vi "0-Load Map.vi"(2 "Map Name":T1="Lake Waban", 3 "Image Ref In":T2) -> (0 "Image Descriptor":T3={"Upper-Left Corner Coordinates"={"UTM Zone"=0.0, "Hemisphere"=enum."North", "East"=0.0, "North"=0.0}, "Meters/Pixel"=1.0} {"Upper-Left Corner Coordinates"."North" format="%#_10f"; "Upper-Left Corner Coordinates"."East" format="%#_8f"}, 1 "Image Ref Out":T2)   [LabVIEW 2011]
doc: "Loads a map and its corresponding descriptor text file.\n\n.png will be added to the given Map Name to get the image,\n.txt will be added to get the image descriptor (The image and the descriptor file have the same filename but different extensions)\nfiles will be retrieved from the /locations/ folder."
uses:
  0-Image Descriptor.ctl
  2-Think/2 Typedefs/UTM Location.ctl
  <vilib>/vision/Image Controls.llb/IMAQ Image.ctl
  0 Typedefs/Maps.ctl
panel:
  # ".png will be added to the map name to get the image,\n.txt will be added to get the image descriptor"
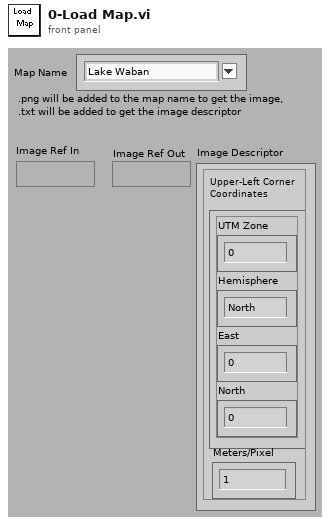
[diagram p1: front panel]
types:
  T1 = typedef "Maps.ctl" = string
  T2 = typedef "IMAQ Image.ctl" = refnum<image>
  T3 = typedef "0-Image Descriptor.ctl" = cluster{"Upper-Left Corner Coordinates":T4, "Meters/Pixel":dbl}
  T4 = typedef "UTM Location.ctl" = cluster{"UTM Zone":dbl, "Hemisphere":enum16{"North", "South"}, "East":dbl, "North":dbl}
  T5 = typedef "Image Type" = u32
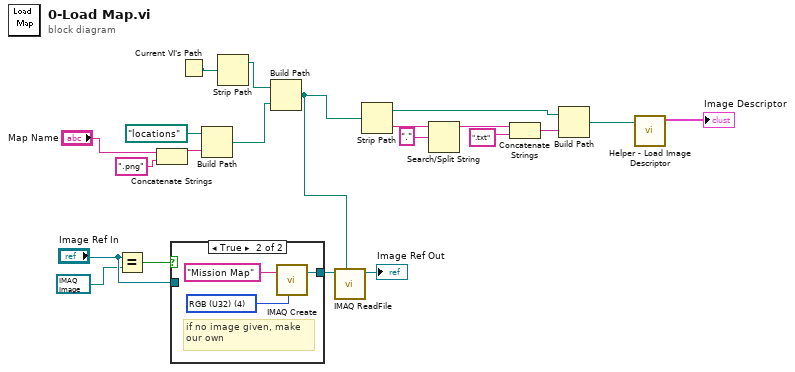
[diagram p0: block diagram]
diagram:
  n1 = Equal?(x="Image Ref In", y=T2 refnum ("Image Ref In 2")) -> (x = y?=w8:bool)
  n2 = Concatenate Strings("Map Name", ".png" ("string")) -> (w6:string)
  n3 = case shown="True" w8 {
    tunnel: [w22 w23] -> w21
    tunnel: "Image Ref In" -> [w22 _]
    frame False {
      # "if image given, use it"
    }
    frame True {
      w24 = T5 4 items=["Grayscale (U8)", "Grayscale (I16)", "Grayscale (SGL)", "Complex (CSG)", "RGB (U32)", "HSL (U32)", "RGB (U64)", "Grayscale (U16)"] ("Image Type")
      # "if no image given, make\nour own"
      n4 = call "IMAQ Create"("Image Name"="Mission Map", "Image Type"=w24) -> ("New Image"=w23:T2)  [unwired: 2 in, 2 out]
    }
  }
  n5 = Current VI's Path() -> (path=w18:path)
  n6 = Build Path(base path=path "locations", name or relative path=w6) -> (appended path=w3:path)
  n7 = Strip Path(path=w18) -> (stripped path=w17:path)  [unwired: 1 out]
  n8 = Build Path(base path=w17, name or relative path=w3) -> (appended path=w9:path)
  n9 = call "IMAQ ReadFile"("File Path"=w9, "Image"=w21) -> ("Image Out"=→"Image Ref Out":T2)  [unwired: 3 in, 6 out]
  n10 = Strip Path(path=w9) -> (stripped path=w12:path, name=w13:string)
  n11 = Search/Split String(string=w13, search string/char (-)=".") -> (substring before match=w14:string)  [unwired: 3 out]
  n12 = Concatenate Strings(w14, ".txt" ("string")) -> (w16:string)
  n13 = Build Path(base path=w12, name or relative path=w16) -> (appended path=w11:path)
  n14 = call "Helper - Load Image Descriptor.vi"("Image Descriptor File Path"=w11) -> ("Image Descriptor Typedef out"=→"Image Descriptor":T3)  [unwired: 10 in]
